vi "set_tree_row.vi"(4 "error in (no error)":errorcluster, 5 "Tag":string, 6 "Row":string[](array[string]), 7 "CtlRef":refnum<vi>) -> (0 "error out":errorcluster, 3 "CtlRef 2":refnum<vi>)   [LabVIEW 2010]
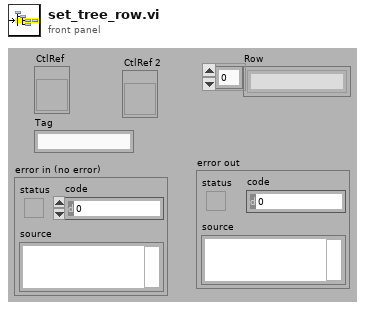
[diagram p1: front panel]
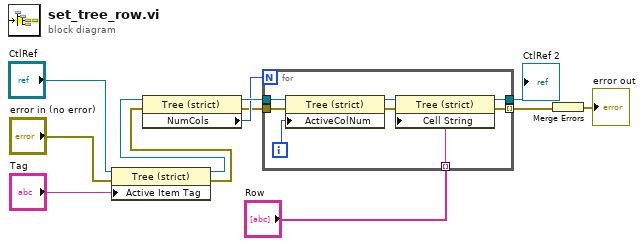
[diagram p0: block diagram]
diagram:
  n1 = property class="Tree (strict)"(reference="CtlRef", error in="error in (no error)", "Active Item Tag"="Tag") -> (reference out=w11:refnum<vi>, error out=w5:errorcluster)
  n2 = property class="Tree (strict)"(reference=w11, error in=w5) -> (reference out=w8:refnum<vi>, error out=w4:errorcluster, "NumCols"=w7:u32)
  n3 = for {
    N: w7 -> [_]
    tunnel: w8 -> [w20]
    tunnel: "Row" -> [w17] mode=indexing
    tunnel: w4 -> [w16]
    tunnel: [w14] -> w2
    tunnel: [w13] -> w3 mode=indexing
    i -> [w18]
    n4 = property class="Tree (strict)"(reference=w20, error in=w16, "ActiveColNum"=w18) -> (reference out=w19:refnum<vi>, error out=w15:errorcluster)
    n5 = property class="Tree (strict)"(reference=w19, error in=w15, "Cell String"=w17) -> (reference out=w14:refnum<vi>, error out=w13:errorcluster)
  }
  "CtlRef 2" <- w2
  n6 = Merge Errors(w3) -> (→"error out":errorcluster)
